vi "New.vi"(5 "FIFO Options":T2, 7 "fifo depths":u32=10, 8 "error in (no error)":errorcluster, 10 "Thread Parameters":T1={"Priority"=100, "Processor"=-2, "ID"=0}, 11 "Plugins":refnum<class "Plugin.lvclass">[](array[class])) -> (0 "error out":errorcluster, 2 "Dispatcher Interface":refnum<class "Dispatcher Interface.lvclass">, 3 "Dispatcher Thread":refnum<class "Dispatcher Thread.lvclass">)   [LabVIEW 2017, in "DSF Core.lvlib" / "Dispatcher Thread.lvclass"]
uses:
  Dispatcher Thread.lvclass
  C:/Users/Admin/Desktop/Data Sharing Framework/Source/Core/Classes/Thread/Thread.lvclass
  Typedefs/DSF FIFO Options.ctl
  Interfaces/Dispatcher/Dispatcher Interface.lvclass
  Thread/Thread Settings.ctl
  Plugin/Plugin.lvclass
  Thread/Thread.lvclass/Thread.ctl
  Dispatcher Thread.lvclass/Dispatcher Thread.ctl
  Thread/Thread.lvclass
  DSF Core.lvlib
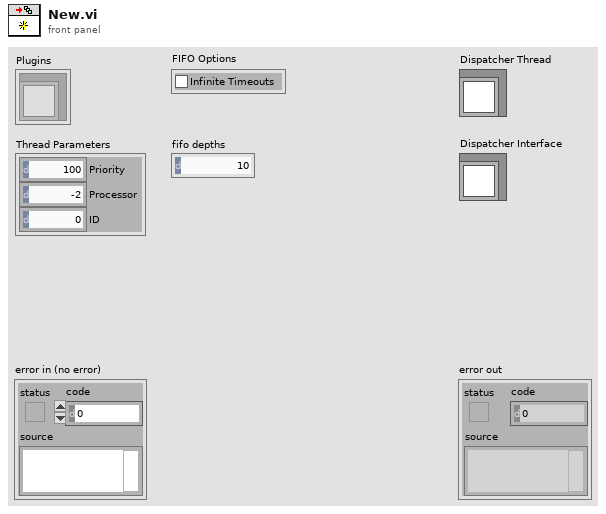
[diagram p1: front panel]
types:
  T1 = typedef "DSF Core.lvlib/Thread.lvclass/Thread Settings.ctl" = cluster{"Priority":u16, "Processor":i32, "ID":i32}
  T2 = typedef "DSF Core.lvlib/DSF FIFO Options.ctl" = cluster{"Infinite Timeouts":bool}
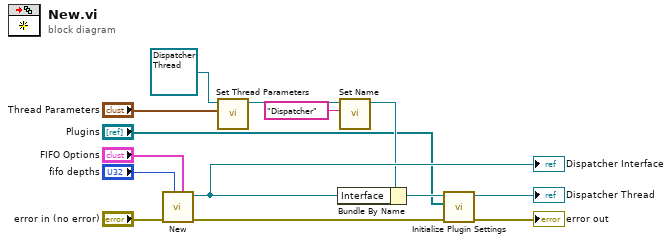
[diagram p0: block diagram]
diagram:
  n1 = call "New.vi"("FIFO Options"="FIFO Options", "fifo depths (10)"="fifo depths", "error in (no error)"="error in (no error)") -> ("error out"=w1:errorcluster, "Dispatcher Interface"=w11:refnum<class "Dispatcher Interface.lvclass">)  [unwired: 7 in]
  "Dispatcher Interface" <- w11
  n2 = call "Set Thread Parameters.vi"("thread settings"="Thread Parameters", "Thread in"=refnum<class "Dispatcher Thread.lvclass"> refnum ("Dispatcher type")) -> ("Thread out"=w8:refnum<class "Dispatcher Thread.lvclass">)  [unwired: 9 in]
  n3 = call "Set Name.vi"("name"="Dispatcher", "Thread in"=w8) -> ("Thread out"=w7:refnum<class "Dispatcher Thread.lvclass">)  [unwired: 9 in]
  n4 = Bundle By Name(cluster=w7, "Interface"=w11) -> (w5:refnum<class "Dispatcher Thread.lvclass">)
  n5 = call "Initialize Plugin Settings.vi"("error in (no error)"=w1, "Plugins"="Plugins", "Dispatcher in"=w5) -> ("error out"=→"error out":errorcluster, "Dispatcher out"=→"Dispatcher Thread":refnum<class "Dispatcher Thread.lvclass">)  [unwired: 7 in]
